vi "Configure for continuous.vi"(7 "Numeric Control":i32=-1, 8 "error in (no error)":errorcluster, 10 "Trigger Timeout (10000000)":dbl=1000.0 format="%#_13g", 11 "Gage digitizer actor in":refnum<class "Gage digitizer actor.lvclass">) -> (0 "error out":errorcluster, 3 "Gage digitizer actor out":refnum<class "Gage digitizer actor.lvclass">)   [LabVIEW 2015]
uses:
  Gage digitizer actor.lvclass
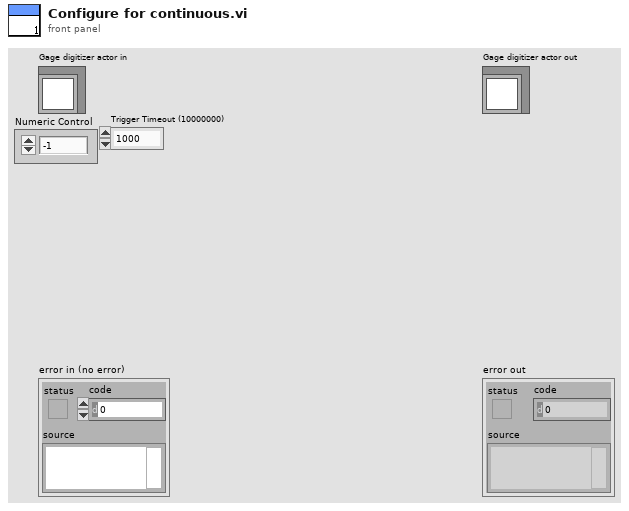
[diagram p1: front panel]
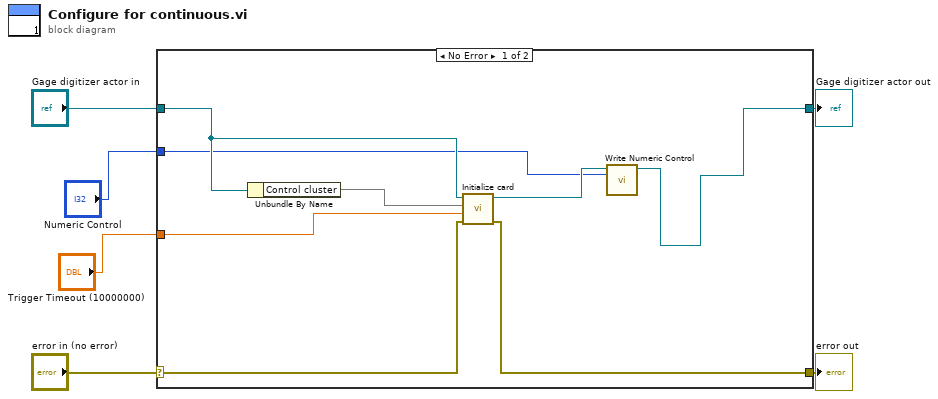
[diagram p0: block diagram]
diagram:
  n1 = case shown="No Error" "error in (no error)" {
    selector: "error in (no error)" -> [w11 w16]
    tunnel: [w10 w16] -> w5
    tunnel: [w8 w15] -> w3
    tunnel: "Gage digitizer actor in" -> [w12 w15]
    tunnel: "Trigger Timeout (10000000)" -> [w13 _]
    tunnel: "Numeric Control" -> [w7 _]
    frame No Error {
      n2 = Unbundle By Name(w12) -> ("Control cluster"=w14)
      n3 = call-dynamic "Initialize card.vi"("error in (no error)"=w11, "Trigger Timeout (10000000)"=w13, "Control cluster"=w14, "Gage digitizer actor in"=w12) -> ("error out"=w10:errorcluster, "Gage digitizer actor out"=w9:refnum<class "Gage digitizer actor.lvclass">)  [unwired: 6 in]
      n4 = call-dynamic "Write Numeric Control.vi"("Numeric Control"=w7, "Gage digitizer actor in"=w9) -> ("Gage digitizer actor out"=w8:refnum<class "Gage digitizer actor.lvclass">)  [unwired: 8 in, 1 out]
    }
    frame Error {
    }
  }
  "error out" <- w5
  "Gage digitizer actor out" <- w3
